vi "Main_Function_VISA.vi"(4 "Delay Time":u32=50, 5 "CRC":bool, 7 "Action_VISA":T1(ring), 8 "Error In":errorcluster, 9 "Comment":string, 10 "VISA Data":T2={"Baud rate"=9600, "Data bits"=8, "Parity"=enum."None", "Stop bits"=10, "Flow control"=0} {"Stop bits" items=["1.0"=10, "1.5"=15, "2.0"=20]; "Flow control" items=["None", "XON/XOFF", "RTS/CTS", "XON/XOFF & RTS/CTS", "DTR/DSR", "XON/XOFF & DTR/DSR"]; "Data bits" min=5 max=8 step=1}, 11 "VISA In":refnum<visa-resource-name>) -> (0 "Error Out":errorcluster, 2 "Response":string, 3 "VISA Out":refnum<visa-resource-name>)   [LabVIEW 2015]
uses:
  <vilib>/Instr/_visa.llb/VISA Configure Serial Port (Instr).vi
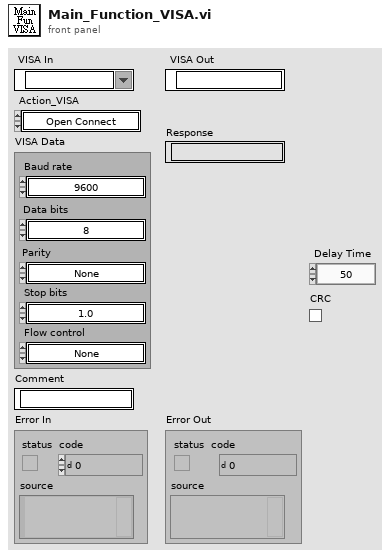
[diagram p1: front panel]
types:
  T1 = enum16{"Open Connect", "Write and Read", "Close Connect"}
  T2 = cluster{"Baud rate":u32, "Data bits":u16, "Parity":enum16{"None", "Odd", "Even", "Mark", "Space"}, "Stop bits":u16, "Flow control":u16}
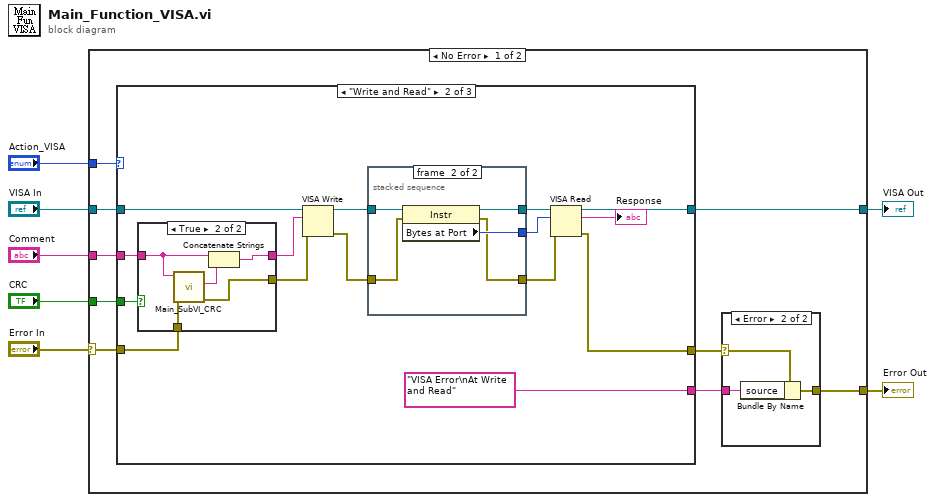
[diagram p0: block diagram]
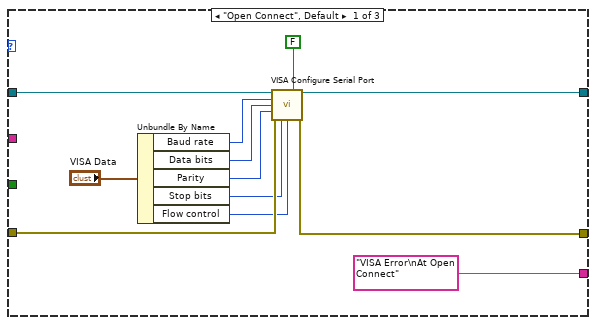
[diagram p3: hidden frame]
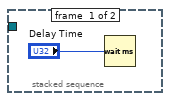
[diagram p4: hidden frame]
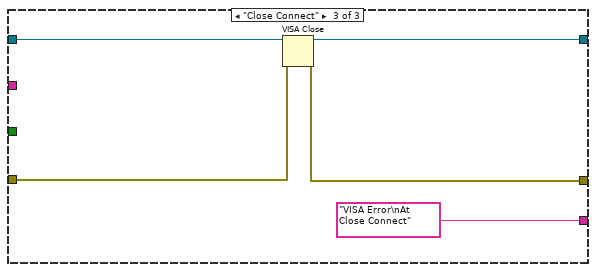
[diagram p6: hidden frame]
diagram:
  n1 = case shown="No Error" "Error In" {
    selector: "Error In" -> [w16 w66]
    tunnel: [w9 w66] -> w6
    tunnel: [w15 w65] -> w5
    tunnel: "Action_VISA" -> [w14 _]
    tunnel: "VISA In" -> [w13 w65]
    tunnel: "Comment" -> [w12 _]
    tunnel: "CRC" -> [w11 _]
    frame No Error {
      n2 = case shown="\"Write and Read\"" w14 {
        tunnel: w16 -> [w30 w44 w64]
        tunnel: [w31 w37 w62] -> w15
        tunnel: [w22 w36 w63] -> w10
        tunnel: w13 -> [w24 w47 w62]
        tunnel: w12 -> [_ w46 _]
        tunnel: w11 -> [_ w45 _]
        tunnel: ["VISA Error\nAt Open Connect" ("source") "VISA Error\nAt Write and Read" ("source") "VISA Error\nAt Close Connect" ("source")] -> w8
        frame "Open Connect", Default {
          n3 = Unbundle By Name("VISA Data") -> ("Baud rate"=w29:u32, "Data bits"=w28:u16, "Parity"=w27:enum16{"None", "Odd", "Even", "Mark", "Space"}, "Stop bits"=w26:u16, "Flow control"=w25:u16)
          n4 = call-poly "VISA Configure Serial Port"("VISA resource name"=w24, "Enable Termination\nChar (T)"=FALSE ("Enable Termination\nChar (T)"), "baud rate (9600)"=w29, "data bits (8)"=w28, "parity (0:none)"=w27, "error in (no error)"=w30, "stop bits (10: 1 bit)"=w26, "flow control (0:none)"=w25) -> ("VISA resource name out"=w31:refnum<visa-resource-name>, "error out"=w22:errorcluster)  [unwired: 6 in]
        }
        frame "Write and Read" {
          n5 = case shown="True" w45 {
            tunnel: w46 -> [w54 w58]
            tunnel: w44 -> [w55 w60]
            tunnel: [w55 w59] -> w43
            tunnel: [w54 w56] -> w35
            frame False {
            }
            frame True {
              n6 = call "Main_SubVI_CRC.vi"("Error In"=w60, "Command"=w58) -> ("Error Out"=w59:errorcluster, "CRC Result"=w57:string)  [unwired: 7 in, 1 out]
              n7 = Concatenate Strings(w58, w57) -> (w56:string)
            }
          }
          n8 = VISA Write(VISA resource name=w47, write buffer=w35, error in (no error)=w43) -> (VISA resource name out=w42:refnum<visa-resource-name>, error out=w39:errorcluster)  [unwired: 1 out]
          n9 = stacked-sequence {
            tunnel: w42 -> [_ w53]
            tunnel: [_ w52] -> w41
            tunnel: [_ w51] -> w40
            tunnel: w39 -> [_ w50]
            tunnel: [_ w49] -> w38
            frame #0 {
              n10 = Wait (ms)(milliseconds to wait="Delay Time") -> ()  [unwired: 1 out]
            }
            frame #1 {
              n11 = property class="Instr"(reference=w53, error in=w50) -> (reference out=w52:refnum<visa-resource-name>, error out=w49:errorcluster, "Bytes at Port"=w51:u32)
            }
          }
          n12 = VISA Read(VISA resource name=w41, byte count=w40, error in (no error)=w38) -> (VISA resource name out=w37:refnum<visa-resource-name>, read buffer=→"Response":string, error out=w36:errorcluster)  [unwired: 1 out]
        }
        frame "Close Connect" {
          n13 = VISA Close(VISA resource name=w62, error in (no error)=w64) -> (error out=w63:errorcluster)
        }
      }
      n14 = case shown="Error" w10 {
        selector: w10 -> [w17 w20]
        tunnel: [w17 w19] -> w9
        tunnel: w8 -> [_ w18]
        frame No Error {
        }
        frame Error {
          n15 = Bundle By Name(cluster=w20, "source"=w18) -> (w19:errorcluster)
        }
      }
    }
    frame Error {
    }
  }
  "Error Out" <- w6
  "VISA Out" <- w5
